vi "boot.vi"(8 "error in (no error)":errorcluster) -> (0 "error out":errorcluster, 3 "FPGA VI Reference Out":refnum<k20>)   [LabVIEW 2018]
uses:
  <vilib>/FPGAPlugInAG/USB-7856R OEM/niLvFpga_Open_USB-7856R OEM.vi
  <vilib>/rvi/interface/common/dynamic/niFpgaDynamicAddResources.vi
  <vilib>/rvi/interface/common/niFpgaWaitOnOcc.vi
  <vilib>/Utility/error.llb/Error Cluster From Error Code.vi
  <vilib>/rvi/errors/niLvFpgaAdjustHostInterfaceError.vi
  <vilib>/rvi/interface/nirviOpenFPGA/nirviOpenFPGA.xnode
  FPGA Bitfiles/PLLsctl_FPGATarget7856_FPGAMaintripleSC_z7MvuiNqZKY.lvbitx
  <vilib>/rvi/interface/nirviMethod/nirviMethod.xnode
  <vilib>/rvi/interface/nirviReadWriteControl/nirviReadWriteControl.xnode
  <vilib>/FPGAPlugInAG/Dynamic/niLvFpga_ConfigureFifo_Dynamic.vi
  <vilib>/rvi/errors/niLvFpgaMergeErrorWithErrorCode.vi
  <vilib>/FPGAPlugInAG/Dynamic/niLvFpga_StartFifo_Dynamic.vi
  <vilib>/rvi/interface/Simulation/niFpgaSimulationCallBeginRW.vi
  <vilib>/FPGAPlugInAG/Dynamic/niLvFpga_ReadFifo_Dynamic.vi
  NiFpgaLv.dll
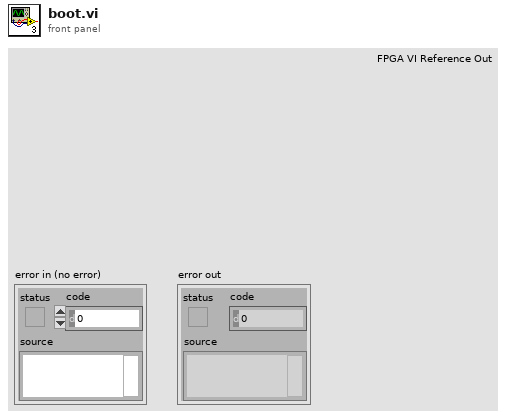
[diagram p1: front panel]
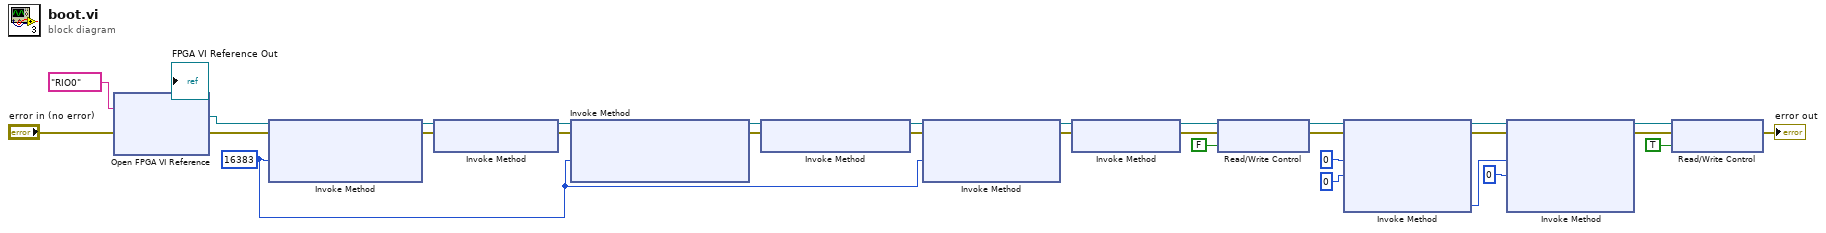
[diagram p0: block diagram]
diagram:
  w2 = u32 16383 ("Requested Depth")
  n1 = xnode "Open FPGA VI Reference"("error in"="error in (no error)", "resource name"=tag "RIO0") -> ("FPGA VI Reference Out"=w1:refnum<k20>, "error out"=w9:errorcluster)
  "FPGA VI Reference Out" <- w1
  n2 = xnode "Invoke Method"("FPGA VI Reference In"=w1, "error in"=w9, "Requested Depth"=w2) -> ("FPGA VI Reference Out"=w7:refnum<k20>, "error out"=w8:errorcluster)  [unwired: 1 out]
  n3 = xnode "Invoke Method"("FPGA VI Reference In"=w7, "error in"=w8) -> ("FPGA VI Reference Out"=w13:refnum<k20>, "error out"=w12:errorcluster)
  n4 = xnode "Invoke Method"("FPGA VI Reference In"=w13, "error in"=w12, "Requested Depth"=w2) -> ("FPGA VI Reference Out"=w10:refnum<k20>, "error out"=w11:errorcluster)  [unwired: 1 out]
  n5 = xnode "Invoke Method"("FPGA VI Reference In"=w10, "error in"=w11) -> ("FPGA VI Reference Out"=w16:refnum<k20>, "error out"=w17:errorcluster)
  n6 = xnode "Invoke Method"("FPGA VI Reference In"=w16, "error in"=w17, "Requested Depth"=w2) -> ("FPGA VI Reference Out"=w14:refnum<k20>, "error out"=w15:errorcluster)  [unwired: 1 out]
  n7 = xnode "Invoke Method"("FPGA VI Reference In"=w14, "error in"=w15) -> ("FPGA VI Reference Out"=w24:refnum<k20>, "error out"=w4:errorcluster)
  n8 = xnode "Read/Write Control"("FPGA VI Reference In"=w24, "error in"=w4, "enable BG log"=FALSE) -> ("FPGA VI Reference Out"=w25:refnum<k20>, "error out"=w28:errorcluster)
  n9 = xnode "Invoke Method"("FPGA VI Reference In"=w25, "error in"=w28, "Number of Elements"=u32 0, "Timeout (ms)"=0) -> ("FPGA VI Reference Out"=w22:refnum<k20>, "error out"=w29:errorcluster, "Elements Remaining"=w23:u32)  [unwired: 1 out]
  n10 = xnode "Invoke Method"("FPGA VI Reference In"=w22, "error in"=w29, "Number of Elements"=w23, "Timeout (ms)"=0) -> ("FPGA VI Reference Out"=w26:refnum<k20>, "error out"=w30:errorcluster)  [unwired: 2 out]
  n11 = xnode "Read/Write Control"("FPGA VI Reference In"=w26, "error in"=w30, "enable BG log"=TRUE) -> ("error out"=→"error out":errorcluster)  [unwired: 1 out]
